vi "GoToTarget.vi"(6 "Extension Power":dbl, 7 "Tolerance Type":T1, 8 "error in (no error)":errorcluster, 9 "target wrist angle (rad; relative to ground)":dbl=nan, 10 "target extension (in.)":dbl=nan, 11 "target arm angle (rad)":dbl=nan) -> (0 "error out":errorcluster, 1 "maxheight":bool[](array[boolean]), 2 "finished":bool, 3 "log":dbl[][](array[numeric]))   [LabVIEW 2014]
uses:
  Robot Global Data.vi
panel:
  in  "Angle tolerance":dbl=5.0 format="%#_13g"
  in  "Extension tolerance":dbl=2.0 format="%#_13g"
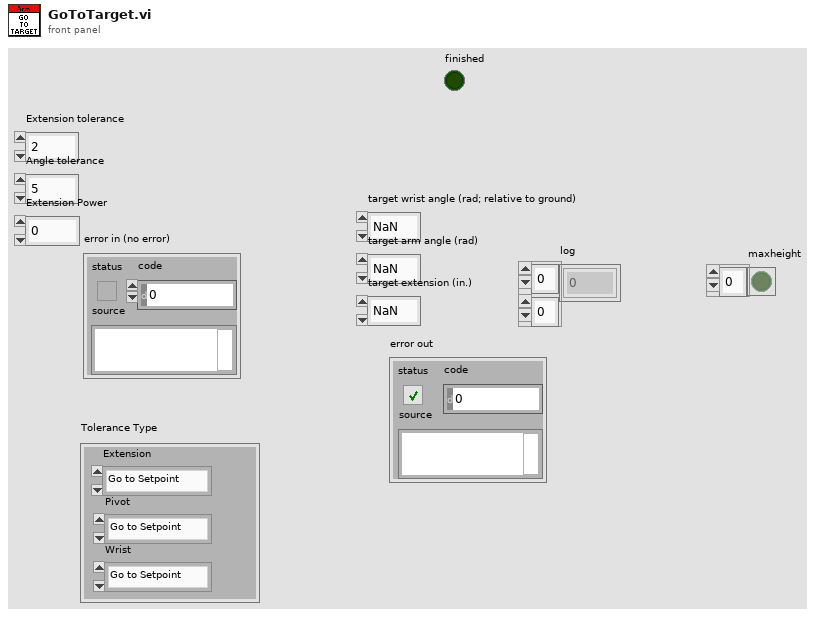
[diagram p1: front panel]
types:
  T1 = cluster{"Extension":enum16{"Go to Setpoint", "Go Past Backward", "Go Past Forward"}, "Pivot":enum16{"Go to Setpoint", "Go Past Backward", "Go Past Forward"}, "Wrist":enum16{"Go to Setpoint", "Go Past Backward", "Go Past Forward"}}
  T2 = typedef "WPI_MotorControlDeviceRef.ctl" = cluster{"DeviceStatus":errorcluster, "Type":T3, "PWM":cluster{"Controller":T4, "PWM Channel":T5, "DeadBand":T6}, "CAN":cluster{"Device Number":u8, "Control Mode":T7, "Semaphore":T8, "Max Vout":dbl, "TalonSRX Control Mode":T9}, "Invert":bool, "TransformRef":T10, "InvTransformRef":T10}
  T3 = typedef "WPI_MotorControlType.ctl" = enum16{"PWM", "CAN", "CANTalonSRX"}
  T4 = typedef "FPGA_TypedefDigitalModule.ctl" = enum16{"Controller 1"}
  T5 = typedef "FPGA_DIOPWMChannel.ctl" = enum8{"PWM 0", "PWM 1", "PWM 2", "PWM 3", "PWM 4", "PWM 5", "PWM 6", "PWM 7", "PWM 8", "PWM 9", "PWM MXP 0", "PWM MXP 1", "PWM MXP 2", "PWM MXP 3", "PWM MXP 4", "PWM MXP 5", "PWM MXP 6", "PWM MXP 7", "PWM MXP 8", "PWM MXP 9", "Invalid"}
  T6 = typedef "WPI_PWMDeadband.ctl" = cluster{"Name":string, "maxPositivePwm":i32, "minPositivePwm":i32, "centerPwm":i32, "maxNegativePwm":i32, "minNegativePwm":i32, "angularRange":u16}
  T7 = typedef "WPI_CANJaguar_ControlMode.ctl" = enum8{"Percent VBus", "Current", "Speed", "Position", "Voltage"}
  T8 = typedef "Semaphore RefNum" = refnum<k1>
  T9 = typedef "WPI_CANTalonSRX_APIControlMode.ctl" = enum8{"Percent VBus", "Speed", "Position", "Slave", "Unchanged / Invalid"}
  T10 = typedef "WPI_PWMTransform_ConPane.ctl" = refnum<vi>
  T11 = enum16{"Go to Setpoint", "Go Past Backward", "Go Past Forward"}
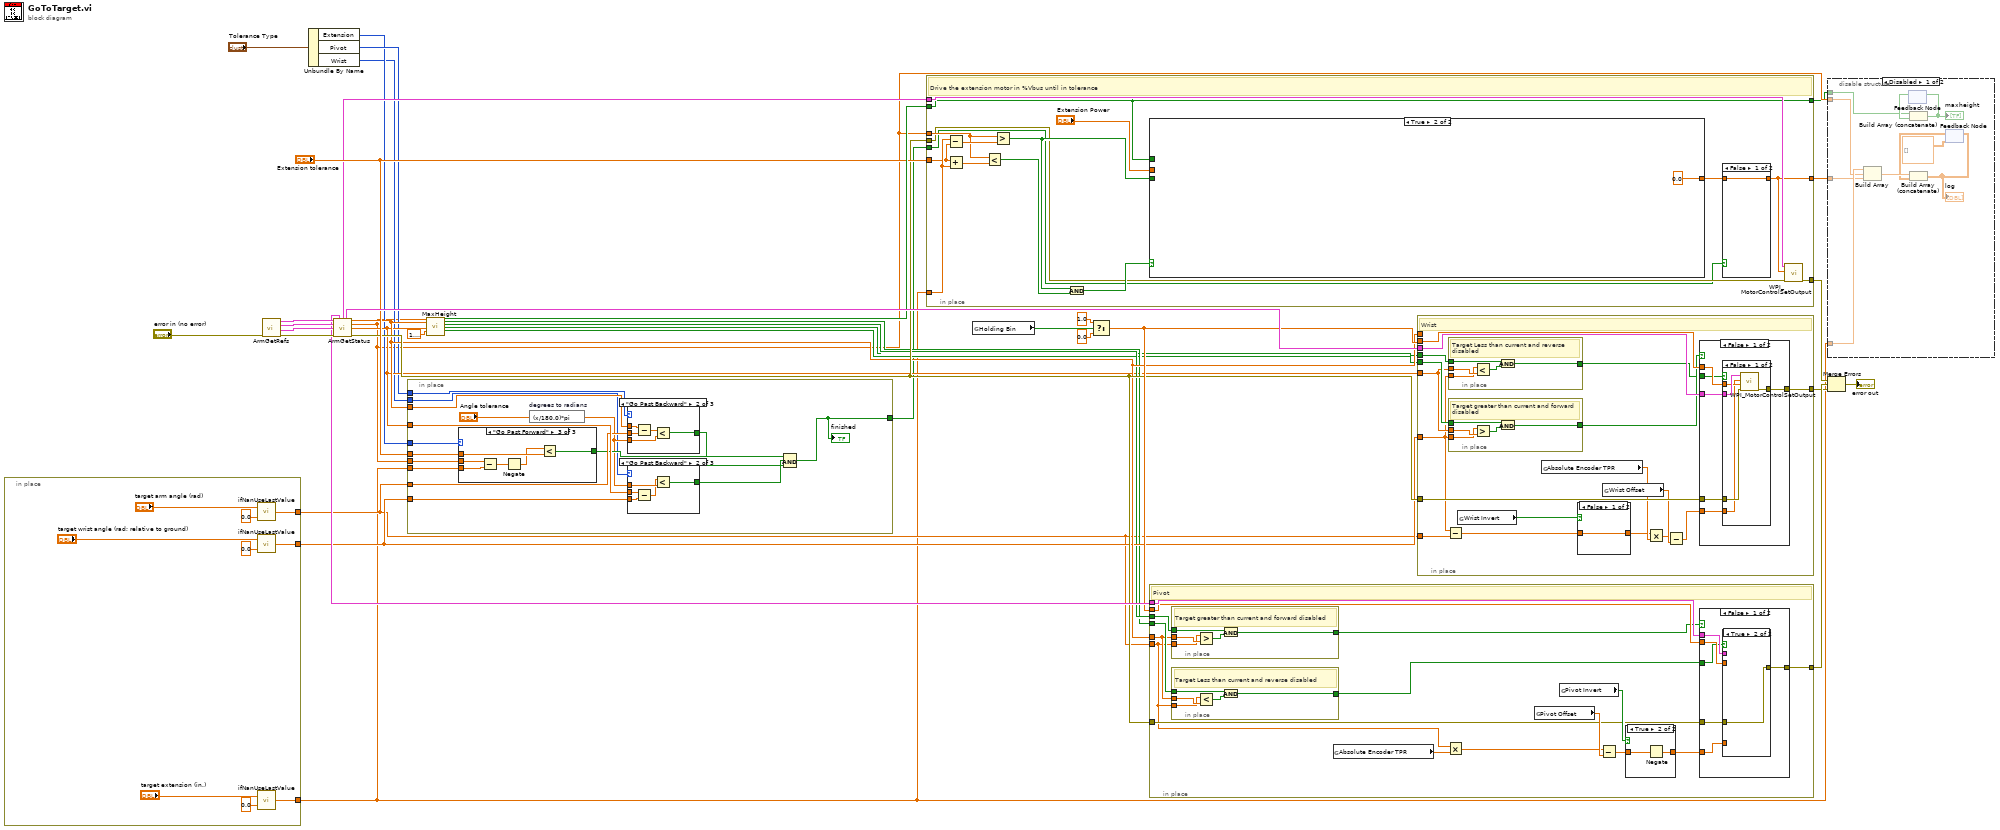
[diagram p0: block diagram]
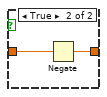
[diagram p5: hidden frame]
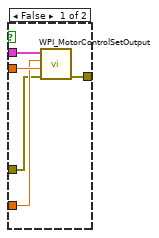
[diagram p6: hidden frame]
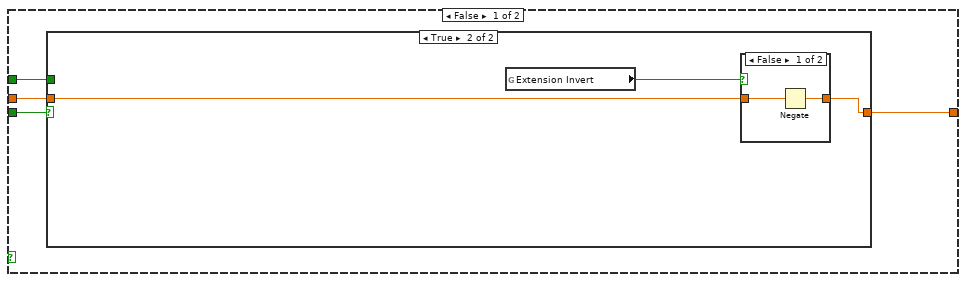
[diagram p10: hidden frame]
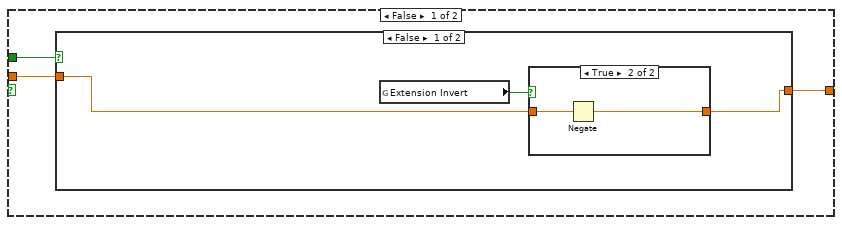
[diagram p11: hidden frame]
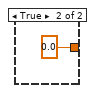
[diagram p13: hidden frame]
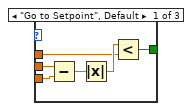
[diagram p15: hidden frame]
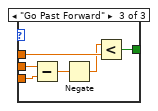
[diagram p16: hidden frame]
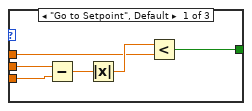
[diagram p17: hidden frame]
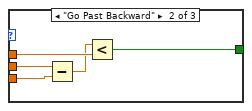
[diagram p18: hidden frame]
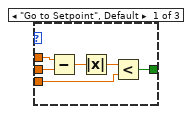
[diagram p19: hidden frame]
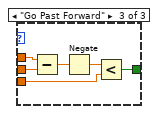
[diagram p20: hidden frame]
diagram:
  n1 = in-place {
    in-place-border: [w41] -> w16
    in-place-border: [w38] -> w6
    in-place-border: [w44] -> w5
    n2 = call "ifNanUseLastValue.vi"("Starting value"=0.0, "Number"="target arm angle (rad)") -> ("Latest num. value"=w38:dbl)
    n3 = call "ifNanUseLastValue.vi"("Starting value"=0.0, "Number"="target wrist angle (rad; relative to ground)") -> ("Latest num. value"=w41:dbl)
    n4 = call "ifNanUseLastValue.vi"("Starting value"=0.0, "Number"="target extension (in.)") -> ("Latest num. value"=w44:dbl)
  }
  n5 = call "ArmGetRefs.vi"("error in (no error)"="error in (no error)") -> ("error out"=w33:errorcluster, "Wrist Ref"=w32:T2, "Extension Ref"=w31:T2, "Pivot Ref"=w30:T2)  [unwired: 7 in]
  n6 = Unbundle By Name("Tolerance Type") -> ("Extension"=w8:T11, "Pivot"=w9:T11, "Wrist"=w7:T11)
  n7 = call "ArmGetStatus.vi"("Pivot Ref"=w30, "ExtensionRef"=w31, "Wrist Ref"=w32, "error in (no error)"=w33) -> ("Pivot Ref out"=w29:T2, "Extension Ref out"=w20:T2, "Wrist Ref out"=w28:T2, "Pivot angle (rad)"=w17:dbl, "Extension (in.)"=w4:dbl, "Wrist angle (rad, relative to ground)"=w11:dbl, "error out"=w19:errorcluster)  [unwired: 3 in, 2 out]
  n8 = in-place {
    in-place-border: w11 -> [w62]
    in-place-border: w16 -> [w61]
    in-place-border: w17 -> [w58]
    in-place-border: w6 -> [w57]
    in-place-border: w4 -> [w56]
    in-place-border: w5 -> [w55]
    in-place-border: "Extension tolerance" -> [w53]
    in-place-border: w9 -> [w52]
    in-place-border: w8 -> [w49]
    in-place-border: w7 -> [w48]
    in-place-border: [w47] -> w1
    n9 = case shown="\"Go Past Forward\"" w49 {
      tunnel: w56 -> [w83 w90 w96]
      tunnel: w55 -> [w82 w89 w95]
      tunnel: [w81 w88 w94] -> w54
      tunnel: w53 -> [w80 w87 w93]
      frame "Go to Setpoint", Default {
        n10 = Subtract(x=w83, y=w82) -> (x-y=w85:dbl)
        n11 = Absolute Value(x=w85) -> (abs(x)=w84:dbl)
        n12 = Less?(x=w84, y=w80) -> (x < y?=w81:bool)
      }
      frame "Go Past Backward" {
        n13 = Subtract(x=w90, y=w89) -> (x-y=w86:dbl)
        n14 = Less?(x=w86, y=w87) -> (x < y?=w88:bool)
      }
      frame "Go Past Forward" {
        n15 = Subtract(x=w96, y=w95) -> (x-y=w92:dbl)
        n16 = Negate(x=w92) -> (-x=w91:dbl)
        n17 = Less?(x=w91, y=w93) -> (x < y?=w94:bool)
      }
    }
    n18 = expression code="(x/180.0)*pi" "degrees to radians"("Angle tolerance") -> (w51:dbl)
    n19 = case shown="\"Go Past Backward\"" w52 {
      tunnel: w58 -> [w101 w107 w113]
      tunnel: w57 -> [w100 w106 w112]
      tunnel: w51 -> [w99 w105 w111]
      tunnel: [w97 w104 w110] -> w50
      frame "Go to Setpoint", Default {
        n20 = Subtract(x=w101, y=w100) -> (x-y=w102:dbl)
        n21 = Absolute Value(x=w102) -> (abs(x)=w98:dbl)
        n22 = Less?(x=w98, y=w99) -> (x < y?=w97:bool)
      }
      frame "Go Past Backward" {
        n23 = Subtract(x=w107, y=w106) -> (x-y=w103:dbl)
        n24 = Less?(x=w103, y=w105) -> (x < y?=w104:bool)
      }
      frame "Go Past Forward" {
        n25 = Subtract(x=w113, y=w112) -> (x-y=w109:dbl)
        n26 = Negate(x=w109) -> (-x=w108:dbl)
        n27 = Less?(x=w108, y=w111) -> (x < y?=w110:bool)
      }
    }
    n28 = case shown="\"Go Past Backward\"" w48 {
      tunnel: w62 -> [w66 w73 w79]
      tunnel: w61 -> [w65 w72 w78]
      tunnel: [w64 w71 w77] -> w60
      tunnel: w51 -> [w63 w70 w76]
      frame "Go to Setpoint", Default {
        n29 = Subtract(x=w66, y=w65) -> (x-y=w68:dbl)
        n30 = Absolute Value(x=w68) -> (abs(x)=w67:dbl)
        n31 = Less?(x=w67, y=w63) -> (x < y?=w64:bool)
      }
      frame "Go Past Backward" {
        n32 = Subtract(x=w73, y=w72) -> (x-y=w69:dbl)
        n33 = Less?(x=w69, y=w70) -> (x < y?=w71:bool)
      }
      frame "Go Past Forward" {
        n34 = Subtract(x=w79, y=w78) -> (x-y=w75:dbl)
        n35 = Negate(x=w75) -> (-x=w74:dbl)
        n36 = Less?(x=w74, y=w76) -> (x < y?=w77:bool)
      }
    }
    n37 = Compound Arithmetic op=AND(w54, w50, w60) -> (w47:bool)
    "finished" <- w47
  }
  n38 = call "MaxHeight.vi"("Extension Length"=w4, "Pivot Angle"=w17, "Wrist Angle (relative to ground)"=w11, "Claw Angle"=1.5707963267948966) -> ("Disable Extend"=w22:bool, "Disable Pivot Reverse"=w14:bool, "Disable Pivot Forward"=w15:bool, "Disable Wrist Reverse"=w12:bool, "Disable Wrist Forward"=w13:bool)  [unwired: 9 in, 2 out]
  n39 = in-place {
    in-place-border: w4 -> [w123]
    in-place-border: w22 -> [w117]
    in-place-border: w5 -> [w122]
    in-place-border: "Extension tolerance" -> [w121]
    in-place-border: w20 -> [w120]
    in-place-border: w19 -> [w119]
    in-place-border: [w118] -> w18
    in-place-border: [w115] -> w3
    in-place-border: [w117] -> w2
    in-place-border: w1 -> [w116]
    # "Drive the extension motor in %Vbus until in tolerance"
    n40 = Subtract(x=w122, y=w121) -> (x-y=w129:dbl)
    n41 = Add(x=w121, y=w122) -> (x+y=w128:dbl)
    n42 = Less?(x=w123, y=w128) -> (x < y?=w127:bool)
    n43 = Greater?(x=w123, y=w129) -> (0:w126:bool)
    n44 = And(x=w126, y=w127) -> (x .and. y?=w124:bool)
    n45 = case shown="True" w124 {
      tunnel: [w133 0.0] -> w114
      tunnel: w126 -> [w134 _]
      tunnel: "Extension Power" -> [w132 _]
      tunnel: w117 -> [w131 _]
      frame False {
        n46 = case shown="True" w134 {
          tunnel: [w136 w145] -> w133
          tunnel: w132 -> [w137 w146]
          tunnel: w131 -> [w135 _]
          frame False {
            n47 = case shown="False" w135 {
              tunnel: w137 -> [w140 _]
              tunnel: [w139 0.0] -> w136
              frame False {
                n48 = global read "Robot Global Data.vi" "Extension Invert"() -> (w138:bool)
                n49 = case shown="True" w138 {
                  tunnel: w140 -> [w141 w143]
                  tunnel: [w141 w142] -> w139
                  frame False {
                  }
                  frame True {
                    n50 = Negate(x=w143) -> (-x=w142:dbl)
                  }
                }
              }
              frame True {
              }
            }
          }
          frame True {
            n51 = global read "Robot Global Data.vi" "Extension Invert"() -> (w147:bool)
            n52 = case shown="False" w147 {
              tunnel: w146 -> [w149 w150]
              tunnel: [w148 w150] -> w145
              frame False {
                n53 = Negate(x=w149) -> (-x=w148:dbl)
              }
              frame True {
              }
            }
          }
        }
      }
      frame True {
      }
    }
    n54 = case shown="False" w116 {
      tunnel: [w130 _] -> w115
      tunnel: w114 -> [w130 _]
      frame False {
      }
      frame True {
      }
    }
    n55 = call <vilib>:"WPI_MotorControlSetOutput.vi"("error in (no error)"=w119, "Output"=w115, "MotorControlDevRef"=w120) -> ("error out"=w118:errorcluster)  [unwired: 6 in, 2 out]
  }
  n56 = global read "Robot Global Data.vi" "Holding Bin"() -> (w27:bool)
  n57 = Select(t=1.0, s=w27, f=0.0) -> (s? t:f=w24:dbl)
  n58 = in-place {
    in-place-border: [w167] -> w37
    in-place-border: w29 -> [w165]
    in-place-border: w24 -> [w161]
    in-place-border: w19 -> [w158]
    in-place-border: w17 -> [w153]
    in-place-border: w6 -> [w152]
    in-place-border: w15 -> [w156]
    in-place-border: w14 -> [w154]
    # "Pivot"
    n59 = in-place {
      in-place-border: [w177] -> w157
      in-place-border: w153 -> [w175]
      in-place-border: w152 -> [w174]
      in-place-border: w156 -> [w173]
      # "Target greater than current and forward disabled"
      n60 = Greater?(x=w174, y=w175) -> (0:w176:bool)
      n61 = And(x=w173, y=w176) -> (x .and. y?=w177:bool)
    }
    n62 = in-place {
      in-place-border: [w172] -> w155
      in-place-border: w153 -> [w170]
      in-place-border: w152 -> [w169]
      in-place-border: w154 -> [w168]
      # "Target Less than current and reverse disabled"
      n63 = Less?(x=w169, y=w170) -> (x < y?=w171:bool)
      n64 = And(x=w168, y=w171) -> (x .and. y?=w172:bool)
    }
    n65 = global read "Robot Global Data.vi" "Absolute Encoder TPR"() -> (w166:dbl)
    n66 = Multiply(x=w152, y=w166) -> (x*y=w163:dbl)
    n67 = global read "Robot Global Data.vi" "Pivot Offset"() -> (w164:dbl)
    n68 = global read "Robot Global Data.vi" "Pivot Invert"() -> (w159:bool)
    n69 = Subtract(x=w163, y=w164) -> (x-y=w162:dbl)
    n70 = case shown="True" w159 {
      tunnel: w162 -> [w191 w193]
      tunnel: [w191 w192] -> w160
      frame False {
      }
      frame True {
        n71 = Negate(x=w193) -> (-x=w192:dbl)
      }
    }
    n72 = case shown="False" w157 {
      tunnel: [w183 w190] -> w167
      tunnel: w165 -> [w182 _]
      tunnel: w161 -> [w181 _]
      tunnel: w160 -> [w180 _]
      tunnel: w158 -> [w179 w190]
      tunnel: w155 -> [w178 _]
      frame False {
        n73 = case shown="True" w178 {
          tunnel: [w188 w189] -> w183
          tunnel: w182 -> [w187 _]
          tunnel: w181 -> [w186 _]
          tunnel: w180 -> [w185 _]
          tunnel: w179 -> [w184 w189]
          frame False {
            n74 = call <vilib>:"WPI_MotorControlSetOutput.vi"("error in (no error)"=w184, "Sync Group / Parameter Slot"=w186, "Output"=w185, "MotorControlDevRef"=w187) -> ("error out"=w188:errorcluster)  [unwired: 5 in, 2 out]
          }
          frame True {
          }
        }
      }
      frame True {
      }
    }
  }
  n75 = in-place {
    in-place-border: [w211] -> w36
    in-place-border: w28 -> [w209]
    in-place-border: w24 -> [w208]
    in-place-border: w19 -> [w207]
    in-place-border: w17 -> [_]
    in-place-border: w16 -> [w195]
    in-place-border: w13 -> [w198]
    in-place-border: w12 -> [w197]
    in-place-border: w11 -> [w196]
    in-place-border: w6 -> [w194]
    # "Wrist"
    n76 = Subtract(x=w195, y=w194) -> (x-y=w210:dbl)
    n77 = in-place {
      in-place-border: [w229] -> w199
      in-place-border: w197 -> [w227]
      in-place-border: w196 -> [w226]
      in-place-border: w195 -> [w225]
      # "Target Less than current and reverse disabled"
      n78 = Less?(x=w225, y=w226) -> (x < y?=w228:bool)
      n79 = And(x=w227, y=w228) -> (x .and. y?=w229:bool)
    }
    n80 = in-place {
      in-place-border: [w234] -> w200
      in-place-border: w198 -> [w232]
      in-place-border: w196 -> [w231]
      in-place-border: w195 -> [w230]
      # "Target greater than current and forward disabled"
      n81 = Greater?(x=w230, y=w231) -> (0:w233:bool)
      n82 = And(x=w232, y=w233) -> (x .and. y?=w234:bool)
    }
    n83 = global read "Robot Global Data.vi" "Wrist Invert"() -> (w201:bool)
    n84 = global read "Robot Global Data.vi" "Absolute Encoder TPR"() -> (w206:dbl)
    n85 = case shown="False" w201 {
      tunnel: w210 -> [w235 w237]
      tunnel: [w235 w236] -> w203
      frame False {
      }
      frame True {
        n86 = Negate(x=w237) -> (-x=w236:dbl)
      }
    }
    n87 = global read "Robot Global Data.vi" "Wrist Offset"() -> (w205:dbl)
    n88 = Multiply(x=w203, y=w206) -> (x*y=w204:dbl)
    n89 = Subtract(x=w204, y=w205) -> (x-y=w202:dbl)
    n90 = case shown="False" w200 {
      tunnel: [w217 w224] -> w211
      tunnel: w209 -> [w216 _]
      tunnel: w208 -> [w215 _]
      tunnel: w207 -> [w214 w224]
      tunnel: w202 -> [w213 _]
      tunnel: w199 -> [w212 _]
      frame False {
        n91 = case shown="False" w212 {
          tunnel: [w222 w223] -> w217
          tunnel: w216 -> [w221 _]
          tunnel: w215 -> [w220 _]
          tunnel: w214 -> [w219 w223]
          tunnel: w213 -> [w218 _]
          frame False {
            n92 = call <vilib>:"WPI_MotorControlSetOutput.vi"("error in (no error)"=w219, "Sync Group / Parameter Slot"=w220, "Output"=w218, "MotorControlDevRef"=w221) -> ("error out"=w222:errorcluster)  [unwired: 5 in, 2 out]
          }
          frame True {
          }
        }
      }
      frame True {
      }
    }
  }
  n93 = disable-structure shown="Disabled" {
    disable-tunnel: w5 -> [w247 _]
    disable-tunnel: w4 -> [w246 _]
    disable-tunnel: w3 -> [w245 _]
    disable-tunnel: w2 -> [w238 _]
    frame Disabled {
      n94 = Build Array(w247, w246, w245) -> (w244:dbl[])
      n95 = feedback #1() -> (w240:bool[])  [unwired: 1 in]
      n96 = Build Array (concatenate)(w238, w240) -> (w239:bool[])
      "maxheight" <- w239
      n97 = feedback-in #1(w239) -> ()
      n98 = feedback #2(dbl[][] [] ("appended array")) -> (w243:dbl[][])
      n99 = Build Array (concatenate)(w244, w243) -> (w241:dbl[][])
      "log" <- w241
      n100 = feedback-in #2(w241) -> ()
    }
    frame Enabled {
    }
  }
  n101 = Merge Errors(w18, w37, w36) -> (→"error out":errorcluster)
